vi "General Cosine Window.vi"   [LabVIEW 2022 SP3, in "NI_AALPro.lvlib"]
doc: "Applies a general cosine window to the input signal <B>X</B>. Wire data to the <B>X</B> input to determine the polymorphic instance to use or manually select the instance."
uses:
  NI_AALPro.lvlib
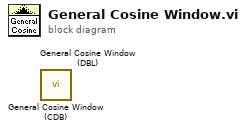
[diagram p0: block diagram]
diagram:
  n1 = call "General Cosine Window (CDB).vi"() -> ()  [unwired: 2 in, 2 out]
  n2 = call "General Cosine Window (DBL).vi"() -> ()  [unwired: 2 in, 2 out]
